vi "stage initialize.vi"(8 "error in":errorcluster, 11 "Combo Box":string(combo)) -> (0 "error out":errorcluster)   [LabVIEW 2015]
uses:
  C:/ProgramData/PI/LabVIEW/Low Level/Communication.llb/Interface Settings.ctl
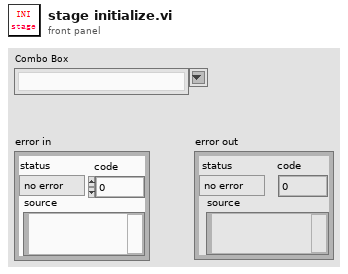
[diagram p1: front panel]
types:
  T1 = typedef "Interface Settings.ctl" = cluster{"Interface":u16, "Timeout":u32, "RS232 settings":cluster{"Portnumber":u8, "Baudrate":u16}, "TCP/IP settings":cluster{"Host address/name":string, "Port":i32, "Board":i32, "TCP/IP Search?":bool}, "USB settings":cluster{"S/N":string, "USB Search?":bool}, "DaisyChain settings":cluster{"Register DC":bool, "DaisyChain Search?":bool, "Device ID":i32}, "DLL for Device":u16}
  T2 = cluster{"Force?":bool, "Dialog?":bool, "Stages":string[]}
  T3 = cluster{"Check FRF?":bool, "Referencing mode":enum16{"FRF (-> FNL)", "FRF", "FNL", "FPL", "RON OFF"}[]}
  T4 = cluster{"RS232 settings":cluster{"Portnumber":i32, "Baudrate":u16}, "USB settings":cluster{"S/N":string, "USB Search?":bool}, "TCP/IP settings":cluster{"Host address/name":string, "Port":i32, "Board":i32, "TCP/IP Search?":bool}}
  T5 = enum16{"Do not reference", "Reference switch", "Negative limit switch", "Positive limit switch"}[]
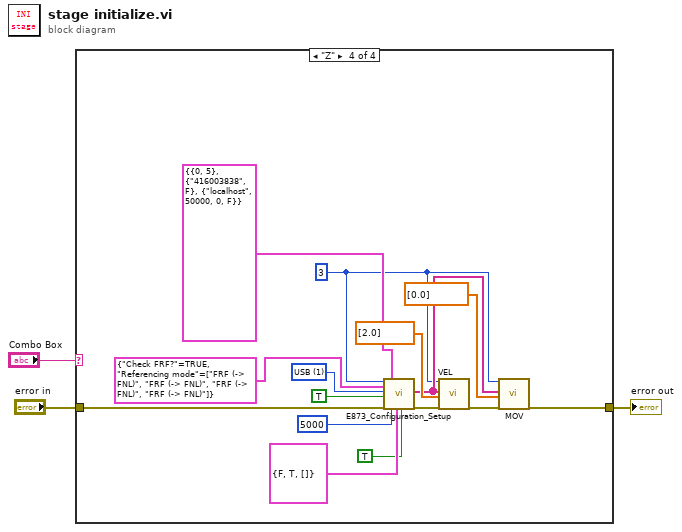
[diagram p0: block diagram]
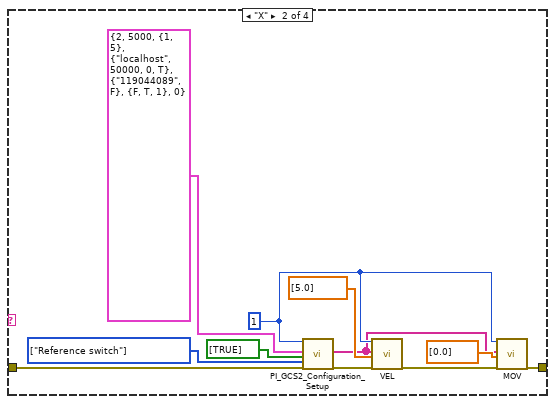
[diagram p3: hidden frame]
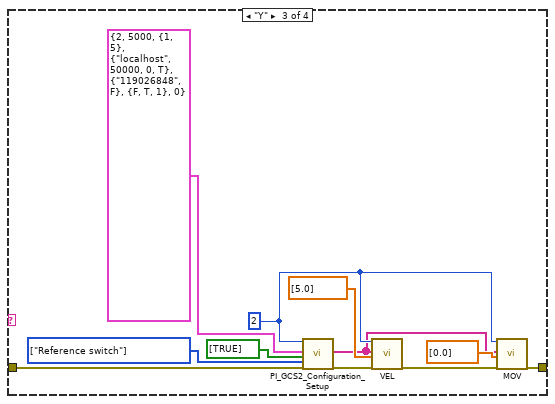
[diagram p4: hidden frame]
diagram:
  n1 = case shown="\"Z\"" "Combo Box" {
    tunnel: "error in" -> [_ w6 w17 w27]
    tunnel: [_ w5 w16 w37] -> w1
    frame "False", Default {
    }
    frame "X" {
      w4 = T5 [enum."Reference switch"] items=["Do not reference", "Reference switch", "Negative limit switch", "Positive limit switch"] ("Reference mode")
      w8 = 1 ("System no.")
      n2 = call "PI_GCS2_Configuration_Setup.vi"("System no."=w8, "Interface settings"=T1 {"Interface"=2, "Timeout"=5000, "RS232 settings"={"Portnumber"=1, "Baudrate"=5}, "TCP/IP settings"={"Host address/name"="localhost", "Port"=50000, "Board"=0, "TCP/IP Search?"=TRUE}, "USB settings"={"S/N"="119044089", "USB Search?"=FALSE}, "DaisyChain settings"={"Register DC"=FALSE, "DaisyChain Search?"=TRUE, "Device ID"=1}, "DLL for Device"=0}, "Closed Loop"=bool[] [TRUE], "Reference mode"=w4, "error in"=w6) -> ("Conn. \nAxes"=w7:string[], "error out"=w9:errorcluster)  [unwired: 3 in, 10 out]
      n3 = call "VEL.vi"("System no."=w8, "Axes to set"=w7, "Velocity values"=dbl[] [5.0], "error in"=w9) -> ("error out"=w11:errorcluster)  [unwired: 2 in, 13 out]
      n4 = call "MOV.vi"("System no."=w8, "Axes to move"=w7, "Position values"=dbl[] [0.0], "error in"=w11) -> ("error out"=w5:errorcluster)  [unwired: 1 in, 14 out]
    }
    frame "Y" {
      w15 = T5 [enum."Reference switch"] items=["Do not reference", "Reference switch", "Negative limit switch", "Positive limit switch"] ("Reference mode")
      w19 = 2 ("System no.")
      n5 = call "PI_GCS2_Configuration_Setup.vi"("System no."=w19, "Interface settings"=T1 {"Interface"=2, "Timeout"=5000, "RS232 settings"={"Portnumber"=1, "Baudrate"=5}, "TCP/IP settings"={"Host address/name"="localhost", "Port"=50000, "Board"=0, "TCP/IP Search?"=TRUE}, "USB settings"={"S/N"="119026848", "USB Search?"=FALSE}, "DaisyChain settings"={"Register DC"=FALSE, "DaisyChain Search?"=TRUE, "Device ID"=1}, "DLL for Device"=0}, "Closed Loop"=bool[] [TRUE], "Reference mode"=w15, "error in"=w17) -> ("Conn. \nAxes"=w18:string[], "error out"=w20:errorcluster)  [unwired: 3 in, 10 out]
      n6 = call "VEL.vi"("System no."=w19, "Axes to set"=w18, "Velocity values"=dbl[] [5.0], "error in"=w20) -> ("error out"=w22:errorcluster)  [unwired: 2 in, 13 out]
      n7 = call "MOV.vi"("System no."=w19, "Axes to move"=w18, "Position values"=dbl[] [0.0], "error in"=w22) -> ("error out"=w16:errorcluster)  [unwired: 1 in, 14 out]
    }
    frame "Z" {
      w35 = u16 1 items=["RS232", "USB", "TCP/IP"] ("Interface")
      w26 = 3 ("System no.")
      n8 = call "E873_Configuration_Setup.vi"("System no."=w26, "Referencing"=T3 {"Check FRF?"=TRUE, "Referencing mode"=[enum."FRF (-> FNL)", enum."FRF (-> FNL)", enum."FRF (-> FNL)", enum."FRF (-> FNL)"]}, "Interface"=w35, "All axes?"=TRUE, "error in"=w27, "Interface settings"=T4 {"RS232 settings"={"Portnumber"=0, "Baudrate"=5}, "USB settings"={"S/N"="416003838", "USB Search?"=FALSE}, "TCP/IP settings"={"Host address/name"="localhost", "Port"=50000, "Board"=0, "TCP/IP Search?"=FALSE}}, "Timeout"=u32 5000, "Stage selection"=T2 {"Force?"=FALSE, "Dialog?"=TRUE, "Stages"=[]}, "Switch servo on?"=TRUE) -> ("Conn. \nAxes"=w29:string[], "error out"=w28:errorcluster)  [unwired: 4 in, 5 out]
      n9 = call "VEL.vi"("System no."=w26, "Axes to set"=w29, "Velocity values"=dbl[] [2.0], "error in"=w28) -> ("error out"=w39:errorcluster)  [unwired: 2 in, 13 out]
      n10 = call "MOV.vi"("System no."=w26, "Axes to move"=w29, "Position values"=dbl[] [0.0], "error in"=w39) -> ("error out"=w37:errorcluster)  [unwired: 1 in, 14 out]
    }
  }
  "error out" <- w1
